vi "Create.vi"(8 "error in (no error)":errorcluster, 9 "# Chans":i32, 10 "Size":i32, 11 "MsgQ":refnum<class "MessageQ.lvclass">) -> (0 "error out":errorcluster, 3 "Data Buffer out":refnum<class "Data Buffer DBL.lvclass">)   [LabVIEW 2020, in "VolatusData.lvlib" / "Data Buffer DBL.lvclass"]
uses:
  Data Buffer DBL.lvclass
  Volatus/MessageQ/MessageQ.lvclass
  Data Buffer DBL.lvclass/Data Buffer DBL.ctl
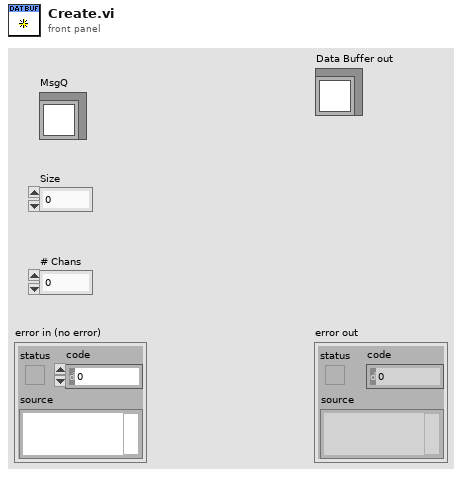
[diagram p1: front panel]
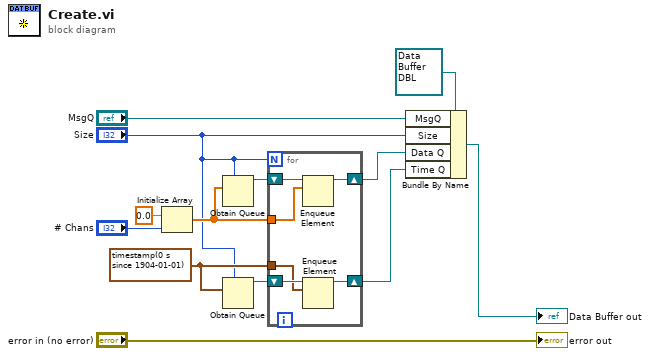
[diagram p0: block diagram]
diagram:
  w4 = timestamp(0 s since 1904-01-01)
  n1 = Initialize Array(0.0 ("element"), "# Chans") -> (w6:dbl[])
  n2 = Obtain Queue(max queue size (-1, unlimited)="Size", element data type=w6) -> (queue out=w10:refnum<queue>)  [unwired: 3 in, 2 out]
  n3 = Obtain Queue(max queue size (-1, unlimited)="Size", element data type=w4) -> (queue out=w5:refnum<queue>)  [unwired: 3 in, 2 out]
  n4 = for {
    N: "Size" -> [_]
    shift-right: [w18] -> w7
    shift-left: w10 -> [w19]
    tunnel: w6 -> [w17]
    tunnel: w4 -> [w15]
    shift-right: [w14] -> w3
    shift-left: w5 -> [w16]
    n5 = Enqueue Element(queue=w19, element=w17) -> (queue out=w18:refnum<queue>)  [unwired: 2 in, 2 out]
    n6 = Enqueue Element(queue=w16, element=w15) -> (queue out=w14:refnum<queue>)  [unwired: 2 in, 2 out]
  }
  n7 = Bundle By Name(cluster=refnum<class "Data Buffer DBL.lvclass"> refnum ("Data Buffer in"), "MsgQ"="MsgQ", "Size"="Size", "Data Q"=w7, "Time Q"=w3) -> (→"Data Buffer out":refnum<class "Data Buffer DBL.lvclass">)
  "error out" <- "error in (no error)"
